vi "GetClassAttributes1.vi"(5 "error in (no error)":errorcluster) -> (12 "created new":bool, 15 "Base class.ClassAttr":i32, 16 "SubClassAttr":i32, 19 "error out":errorcluster)   [LabVIEW 2010, in "G#SubClass2.lvclass"]
uses:
  G#SubClass2.lvclass
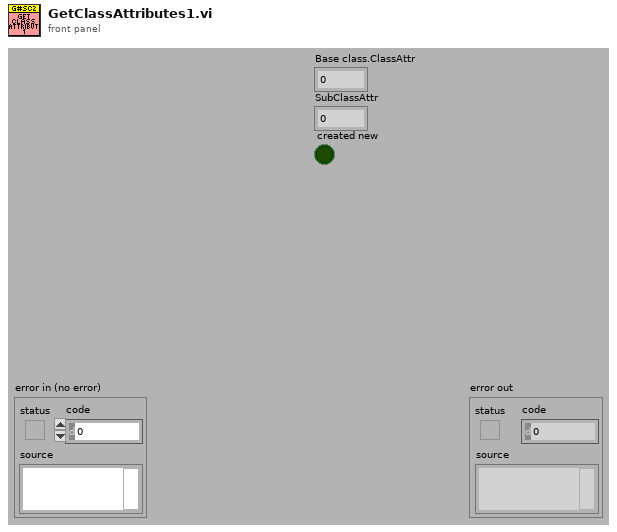
[diagram p1: front panel]
types:
  T1 = typedef "G#SubClass2.lvclass/ClassAttributes.ctl" = cluster{"Base class":T2, "SubClassAttr":i32}
  T2 = typedef "G#BaseClass2.lvclass/ClassAttributes.ctl" = cluster{"ClassAttr":i32}
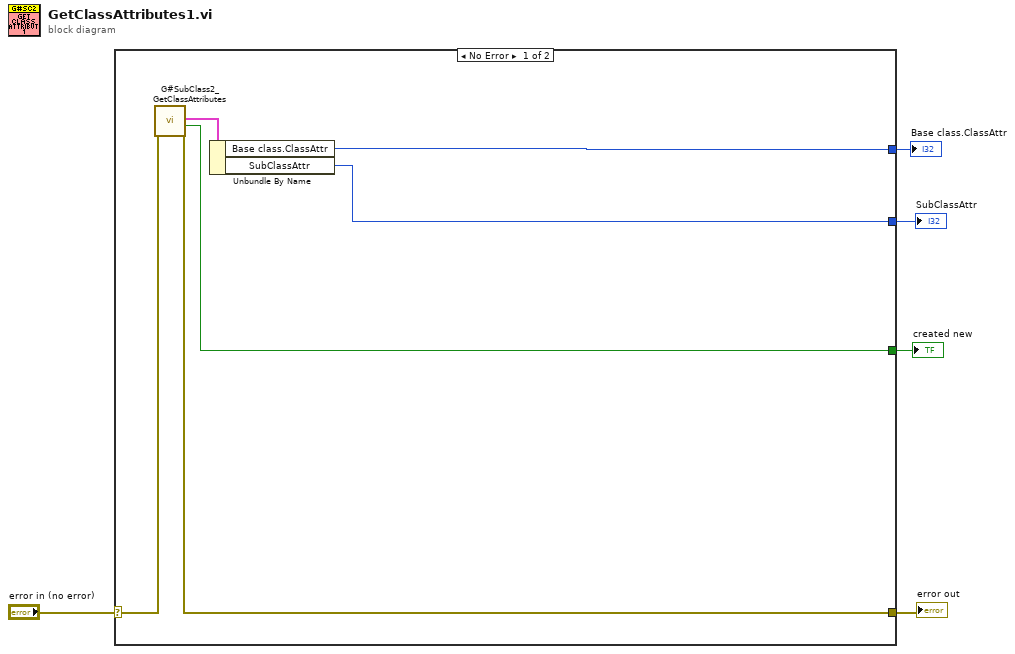
[diagram p0: block diagram]
diagram:
  n1 = case shown="No Error" "error in (no error)" {
    selector: "error in (no error)" -> [w11 w12]
    tunnel: [w10 w12] -> w4
    tunnel: [w8 _] -> w3
    tunnel: [w7 _] -> w2
    tunnel: [w6 _] -> w1
    frame No Error {
      n2 = call "G#SubClass2_GetClassAttributes.vi"("error in (no error)"=w11) -> ("class attributes"=w9:T1, "created new"=w6:bool, "error out"=w10:errorcluster)  [unwired: 14 in, 2 out]
      n3 = Unbundle By Name(w9) -> ("Base class.ClassAttr"=w8:i32, "SubClassAttr"=w7:i32)
    }
    frame Error {
    }
  }
  "error out" <- w4
  "Base class.ClassAttr" <- w3
  "SubClassAttr" <- w2
  "created new" <- w1
